vi "Deserialise content.vi"(8 "error in (no error)":errorcluster, 10 "JSON String to decode":string, 11 "object in":refnum<class "inspect_reply Message.lvclass">) -> (0 "error out":errorcluster, 3 "object out":refnum<class "inspect_reply Message.lvclass">)   [LabVIEW 2018, in "ClientMessaging.lvlib" / "inspect_reply Message.lvclass"]
uses:
  inspect_reply Message.lvclass
  C:/Users/gavin/Documents/LabVIEW Data/LabVIEW-Bits/Connectivity/Jupyter Client/Base Classes/Reply Message/Reply Message.lvclass
  inspect_reply Message.lvclass/inspect_reply Message.ctl
  15a8157c-1e78-44af-b4bc-6bda108fd11f.vi
  4a30924a-ee89-4ed8-ba26-4bd9383c51d3.vi
  753dac7b-068b-4d38-91b4-04c5bbc1270a.vi
  15a8157c-1e78-44af-b4bc-6bda108fd11f.vi/8c3bf01e-ceee-4823-b8fc-3e039343bf83.vi
  15a8157c-1e78-44af-b4bc-6bda108fd11f.vi/02ba5cfa-b8e4-4c34-8170-5d85b6254663.vi
  4a30924a-ee89-4ed8-ba26-4bd9383c51d3.vi/4a8d8b1a-177e-4b5a-870b-adbd9542ac65.vi
  4a30924a-ee89-4ed8-ba26-4bd9383c51d3.vi/de89588e-71f3-434d-a226-4c94648f2a3a.vi
  753dac7b-068b-4d38-91b4-04c5bbc1270a.vi/af3fb89b-2173-4618-b9cc-a5eec191d621.vi
  753dac7b-068b-4d38-91b4-04c5bbc1270a.vi/08bf3e05-07aa-434a-a15b-7ca90501653f.vi
  <userlib>/_OpenG.lib/lvdata/lvdata.llb/Get Cluster Element by Name__ogtk.vi
  Base Classes/Message Class/Message Class.lvclass
  Base Classes/Reply Message/Reply Message.lvclass
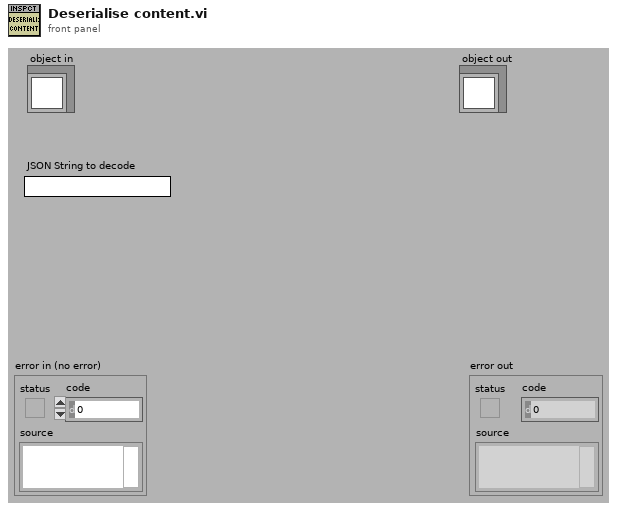
[diagram p1: front panel]
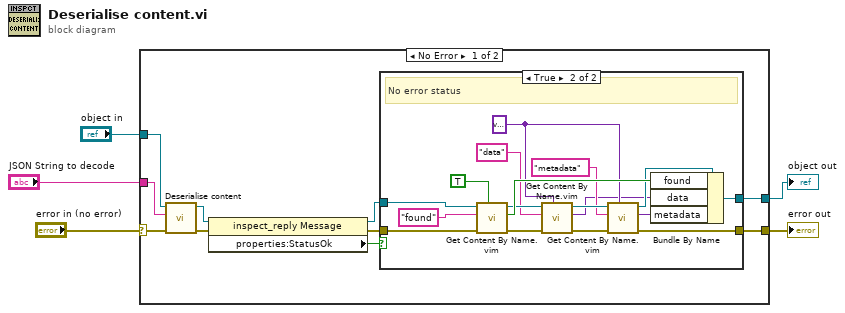
[diagram p0: block diagram]
diagram:
  n1 = case shown="No Error" "error in (no error)" {
    selector: "error in (no error)" -> [w12 w36]
    tunnel: [w6 w36] -> w4
    tunnel: [w8 w35] -> w2
    tunnel: "object in" -> [w15 w35]
    tunnel: "JSON String to decode" -> [w13 _]
    frame No Error {
      n2 = call-parent "Deserialise content.vi"("error in (no error)"=w12, "JSON String to decode"=w13, "object in"=w15) -> ("error out"=w11:errorcluster, "object out"=w14:refnum<class "inspect_reply Message.lvclass">)  [unwired: 7 in]
      n3 = property class="inspect_reply Message"(reference=w14, error in=w11) -> (reference out=w7:refnum<class "inspect_reply Message.lvclass">, error out=w9:errorcluster, "properties:StatusOk"=w10:bool)
      n4 = case shown="True" w10 {
        tunnel: w7 -> [w16 w33]
        tunnel: w9 -> [w17 w32]
        tunnel: [w16 w34] -> w8
        tunnel: [w17 w19] -> w6
        frame False {
          # "error status handled in parent class"
        }
        frame True {
          w22 = variant
          # "No error status"
          n5 = call "Get Content By Name.vim"("Type of content"=TRUE, "error in (no error)"=w32, "Name of Content Item"="found" ("Element Name"), "Message In"=w33) -> ("error out"=w27:errorcluster, "Data Out"=w29:bool, "Message Out"=w28:refnum<class "inspect_reply Message.lvclass">)  [unwired: 5 in]
          n6 = call "Get Content By Name.vim"("Type of content"=w22, "error in (no error)"=w27, "Name of Content Item"="data" ("Element Name"), "Message In"=w28) -> ("error out"=w24:errorcluster, "Data Out"=w18:variant, "Message Out"=w25:refnum<class "inspect_reply Message.lvclass">)  [unwired: 5 in]
          n7 = call "Get Content By Name.vim"("Type of content"=w22, "error in (no error)"=w24, "Name of Content Item"="metadata" ("Element Name"), "Message In"=w25) -> ("error out"=w19:errorcluster, "Data Out"=w21:variant, "Message Out"=w20:refnum<class "inspect_reply Message.lvclass">)  [unwired: 5 in]
          n8 = Bundle By Name(cluster=w20, "found"=w29, "data"=w18, "metadata"=w21) -> (w34:refnum<class "inspect_reply Message.lvclass">)
        }
      }
    }
    frame Error {
    }
  }
  "error out" <- w4
  "object out" <- w2
